vi "Parse Arguments.vi"(8 "error in (no error)":errorcluster, 9 "Args":string[](array[string]), 10 "Folder":path, 11 "InitAction in":refnum<class "InitAction.lvclass">) -> (0 "error out":errorcluster, 3 "InitAction out":refnum<class "InitAction.lvclass">)   [LabVIEW 2020, in "GPackTools.lvlib" / "InitAction.lvclass"]
uses:
  InitAction.lvclass
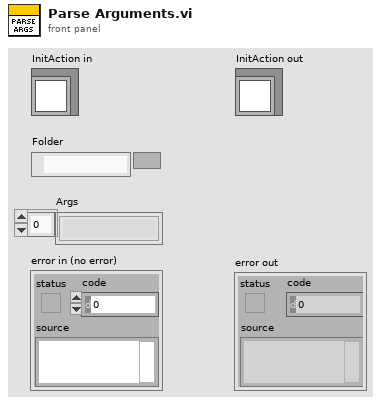
[diagram p1: front panel]
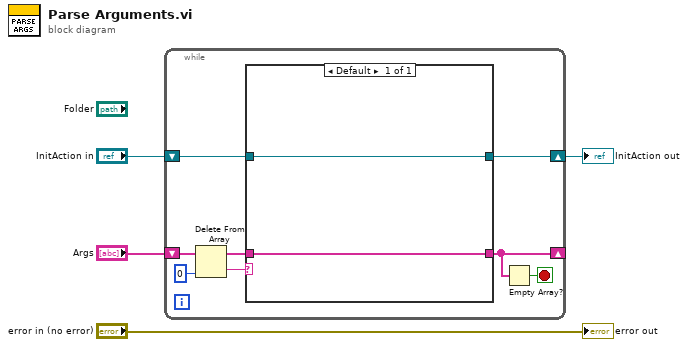
[diagram p0: block diagram]
diagram:
  n1 = while {
    shift-right: [w5] -> w1
    shift-left: "InitAction in" -> [w6]
    shift-right: [w8] -> _
    shift-left: "Args" -> [w12]
    stop <- w7 stop-if-true
    n2 = Delete From Array(array=w12, index=0) -> (deleted portion=w10:string, array with subset deleted=w9:string[])  [unwired: 1 in]
    n3 = case shown="Default" w10 {
      tunnel: w9 -> [w14]
      tunnel: [w14] -> w8
      tunnel: w6 -> [w13]
      tunnel: [w13] -> w5
      frame Default {
      }
    }
    n4 = Empty Array?(array=w8) -> (empty?=w7:bool)
  }
  "InitAction out" <- w1
  "error out" <- "error in (no error)"
